vi "Update Property.vi"(8 "error in (no error)":errorcluster, 9 "Value":variant, 10 "Name":string, 11 "TextPanel in":refnum<class "TextPanel.lvclass">) -> (0 "error out":errorcluster, 3 "TextPanel out":refnum<class "TextPanel.lvclass">)   [LabVIEW 2020, in "Conditum-Tools.lvlib" / "TextPanel.lvclass"]
uses:
  TextPanel.lvclass
  TextPanel.lvclass/TextPanel.ctl
  Conditum-Clone/Columns/Text/Text.lvclass
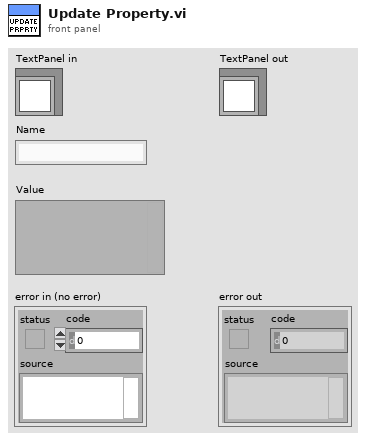
[diagram p1: front panel]
types:
  T1 = typedef "Conditu2.lvlib/Columns.lvlib/Text.lvclass/Definition.ctl" = cluster{"Default":string}
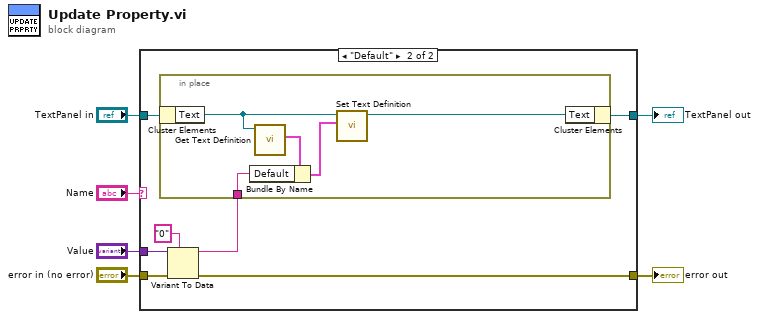
[diagram p0: block diagram]
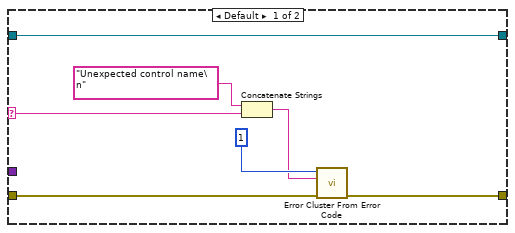
[diagram p2: hidden frame]
diagram:
  n1 = case shown="\"Default\"" "Name" {
    selector: "Name" -> [w9 _]
    tunnel: "Value" -> [_ w20]
    tunnel: "TextPanel in" -> [w7 w16]
    tunnel: "error in (no error)" -> [w13 w18]
    tunnel: [w12 w17] -> w4
    tunnel: [w7 w14] -> w3
    frame Default {
      n2 = Concatenate Strings("Unexpected control name\n" ("format string"), w9) -> (w8:string)
      n3 = call <vilib>:"Error Cluster From Error Code.vi"("error in (no error)"=w13, "error message (\"\")"=w8, "error code (0)"=1) -> ("error out"=w12:errorcluster)  [unwired: 6 in]
    }
    frame "Default" {
      n4 = Variant To Data(error in=w18, type="0", Variant=w20) -> (data=w15:string, error out=w17:errorcluster)
      n5 = in-place {
        in-place-border: w15 -> [w24]
        n6 = in-place-cluster #1(w16) -> ("Text"=w23:refnum<class "Text.lvclass">)
        n7 = call "Get Text Definition.vi"("Text in"=w23) -> ("Definition"=w25:T1)  [unwired: 10 in]
        n8 = Bundle By Name(cluster=w25, "Default"=w24) -> (w22:T1)
        n9 = call "Set Text Definition.vi"("Text Definition"=w22, "Text in"=w23) -> ("Text out"=w21:refnum<class "Text.lvclass">)  [unwired: 9 in]
        n10 = in-place-cluster #1("Text"=w21) -> (w14:refnum<class "TextPanel.lvclass">)
      }
    }
  }
  "error out" <- w4
  "TextPanel out" <- w3
